vi "Init.vi"(8 "error in (no error)":errorcluster, 10 "Instrument Ref":variant, 11 "Keysight 6700C in":refnum<class "Keysight 6700C.lvclass">) -> (0 "error out":errorcluster, 2 "Found?":bool, 3 "Keysight 6700C out":refnum<class "Keysight 6700C.lvclass">)   [LabVIEW 2025, in "Power Supply.lvlib" / "Keysight 6700C.lvclass"]
uses:
  Keysight 6700C.lvclass
  Users/Public/Documents/Sandia National Labs/TSS Plugin/Abstract Engine.lvlibp/Plugin/Abstract/Instrument configuration/Instrument configuration.lvclass
  Keysight 6700C.lvclass/Keysight 6700C.ctl
  Users/Public/Documents/Sandia National Labs/TSS Plugin/Abstract Engine.lvlibp/Plugin/Abstract/Instrument configuration/Read Instrument Setting.vi
  Users/Public/Documents/Sandia National Labs/TSS Plugin/CEF.lvlibp/serializable configuration/CEF_serializable configuration.lvclass
  <instrlib>/Agilent N6700 Series/Agilent N6700 Series.lvlib
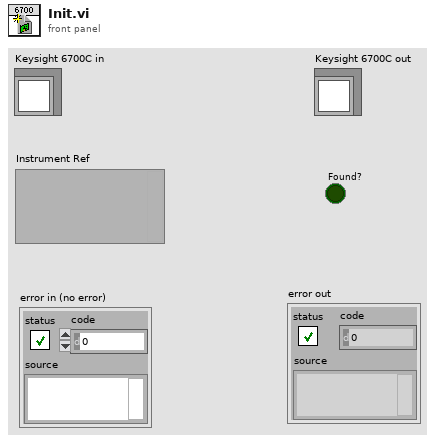
[diagram p1: front panel]
types:
  T1 = typedef "Abstract Engine.lvlibp/Instrument configuration.lvclass/Default Instrument.ctl" = cluster{"Type":string, "Address":string, "SW Alias":string, "Description":string, "Enabled":bool}
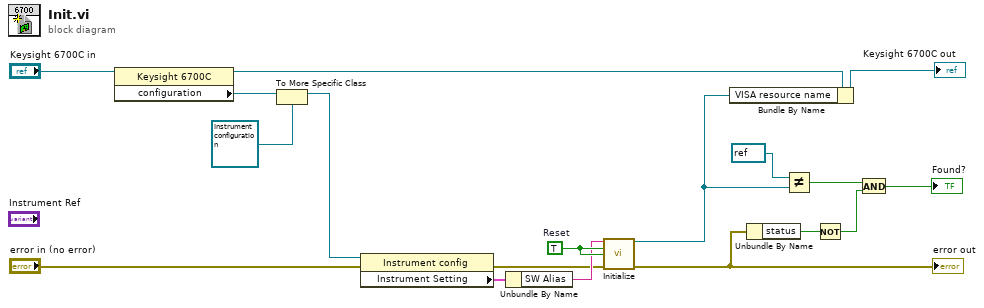
[diagram p0: block diagram]
diagram:
  w18 = TRUE  # Reset
  n1 = property class="Keysight 6700C"(reference="Keysight 6700C in") -> (reference out=w11:refnum<class "Keysight 6700C.lvclass">, "configuration"=w14:refnum<class "CEF_serializable configuration.lvclass">)  [unwired: 1 in, 1 out]
  n2 = To More Specific Class(target class=refnum<class "Instrument configuration.lvclass"> refnum ("Abstract PlugIn.lvlibp:Instrument configuration"), reference=w14) -> (specific class reference=w15:refnum<class "Instrument configuration.lvclass">)  [unwired: 1 in, 1 out]
  n3 = property class="Instrument config"(reference=w15, error in="error in (no error)") -> (error out=w8:errorcluster, "Instrument Setting"=w1:T1)  [unwired: 1 out]
  n4 = Unbundle By Name(w1) -> ("SW Alias"=w12:string)
  n5 = call <instrlib>:"Initialize.vi"("VISA resource name"=w12, "ID Query? (T: Yes)"=w18, "Reset? (T: Yes)"=w18, "error in (no error)"=w8) -> ("VISA resource name out"=w16:refnum<visa-resource-name>, "error out"=w6:errorcluster)  [unwired: 10 in]
  "error out" <- w6
  n6 = Bundle By Name(cluster=w11, "VISA resource name"=w16) -> (→"Keysight 6700C out":refnum<class "Keysight 6700C.lvclass">)
  n7 = Unbundle By Name(w6) -> ("status"=w7:bool)
  n8 = Not Equal?(x=refnum<visa-resource-name> refnum ("VISA resource name out"), y=w16) -> (x != y?=w5:bool)
  n9 = Not(x=w7) -> (.not. x?=w4:bool)
  n10 = And(x=w5, y=w4) -> (x .and. y?=→"Found?":bool)
